vi "Close.vi"(8 "Error In":errorcluster, 11 "Leap Handle":T1) -> (0 "Error Out":errorcluster)   [LabVIEW 2014]
doc: "Close the connection to the Leap Controller."
uses:
  Typedef 2.0/Leap Handle.ctl
  C:/Users/Frax/Desktop/Progetti avanzati Labview/Smart Wristband/Smart Wristband/Leap Motion VIs 2.0/LeapCSharp.NET4.0.dll
  LeapCSharp.NET4.0.dll
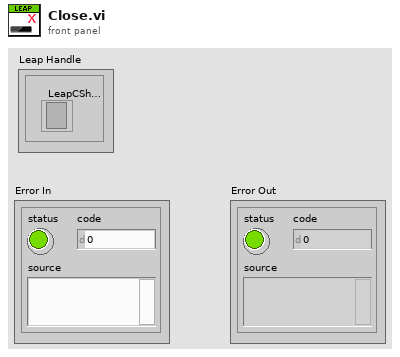
[diagram p1: front panel]
types:
  T1 = typedef "Leap Handle.ctl" = cluster{"LeapCSharp":refnum<k24>}
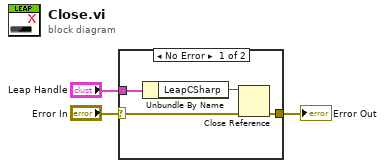
[diagram p0: block diagram]
diagram:
  n1 = case shown="No Error" "Error In" {
    selector: "Error In" -> [w4 w8]
    tunnel: [w6 w8] -> w2
    tunnel: "Leap Handle" -> [w7 _]
    frame No Error {
      n2 = Unbundle By Name(w7) -> ("LeapCSharp"=w5:refnum<k24>)
      n3 = Close Reference(reference=w5, error in (no error)=w4) -> (error out=w6:errorcluster)
    }
    frame Error {
    }
  }
  "Error Out" <- w2
